vi "MonitoringOK7Param-moche.vi"() -> ()   [LabVIEW 2013]
panel:
  in  "Envoi":bool
  in  "data in":string
  out "?":bool
  in  "Afficher caractères reçus":bool
  in  "Log":bool
  out "error out":errorcluster
  out "Caractères reçus":string
  in  "Mode":T1(ring)=enum."CRLF"
  in  "?":bool
  in  "Tab Control":T2(tab)
  out "Par2":dbl
  out "Par1":dbl
  out "Signal Camera     ->    Fronts détectés":dbl[](graph)
  out "Signal Camera    ->  original":dbl[](graph)
  out "Par3":dbl
  out "Par 4":dbl
  out "Par 5":dbl
  out "Par 6":dbl
  out "Par 7":dbl
  in  "PID 3.3":dbl
  in  "PID 3.2":dbl
  in  "PID Direction":dbl
  in  "ABS":bool
  out "?":bool
  in  "PID vitesse":bool
  out "?":bool
  out "?":bool
  in  "PID 2.3":i8
  in  "PID 2.2":i8
  in  "PID Léger":i8
  in  "PID 1.3":i8
  in  "PID 1.2":i8
  in  "PID Fort":i8
  # "Fort"
  # "Léger"
  # "Droite"
  # "Gauche"
  # "Fin"
  # "Perte Ligne"
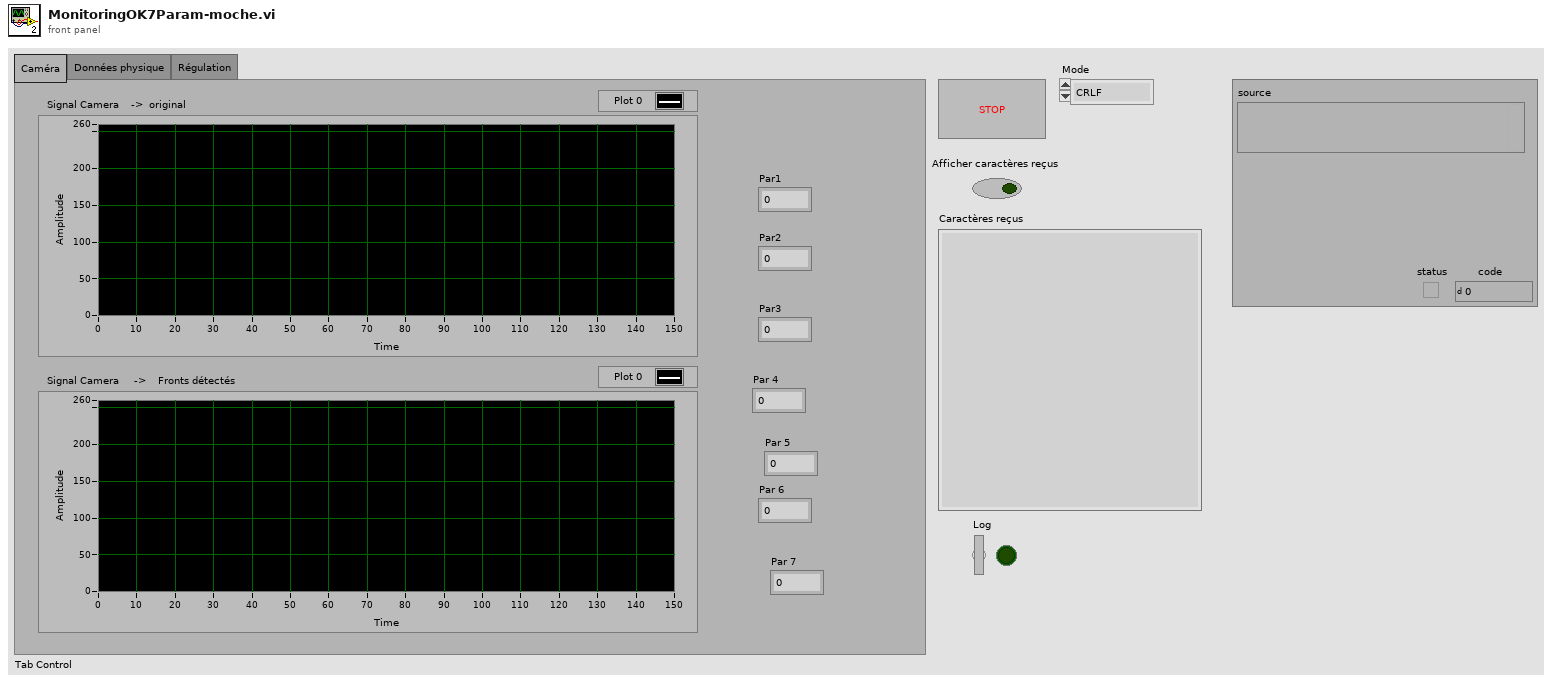
[diagram p1: front panel]
types:
  T1 = enum16{"Standard", "Buffered", "CRLF", "Immediate"}
  T2 = enum32{"Caméra", "Données physique", "Régulation"}
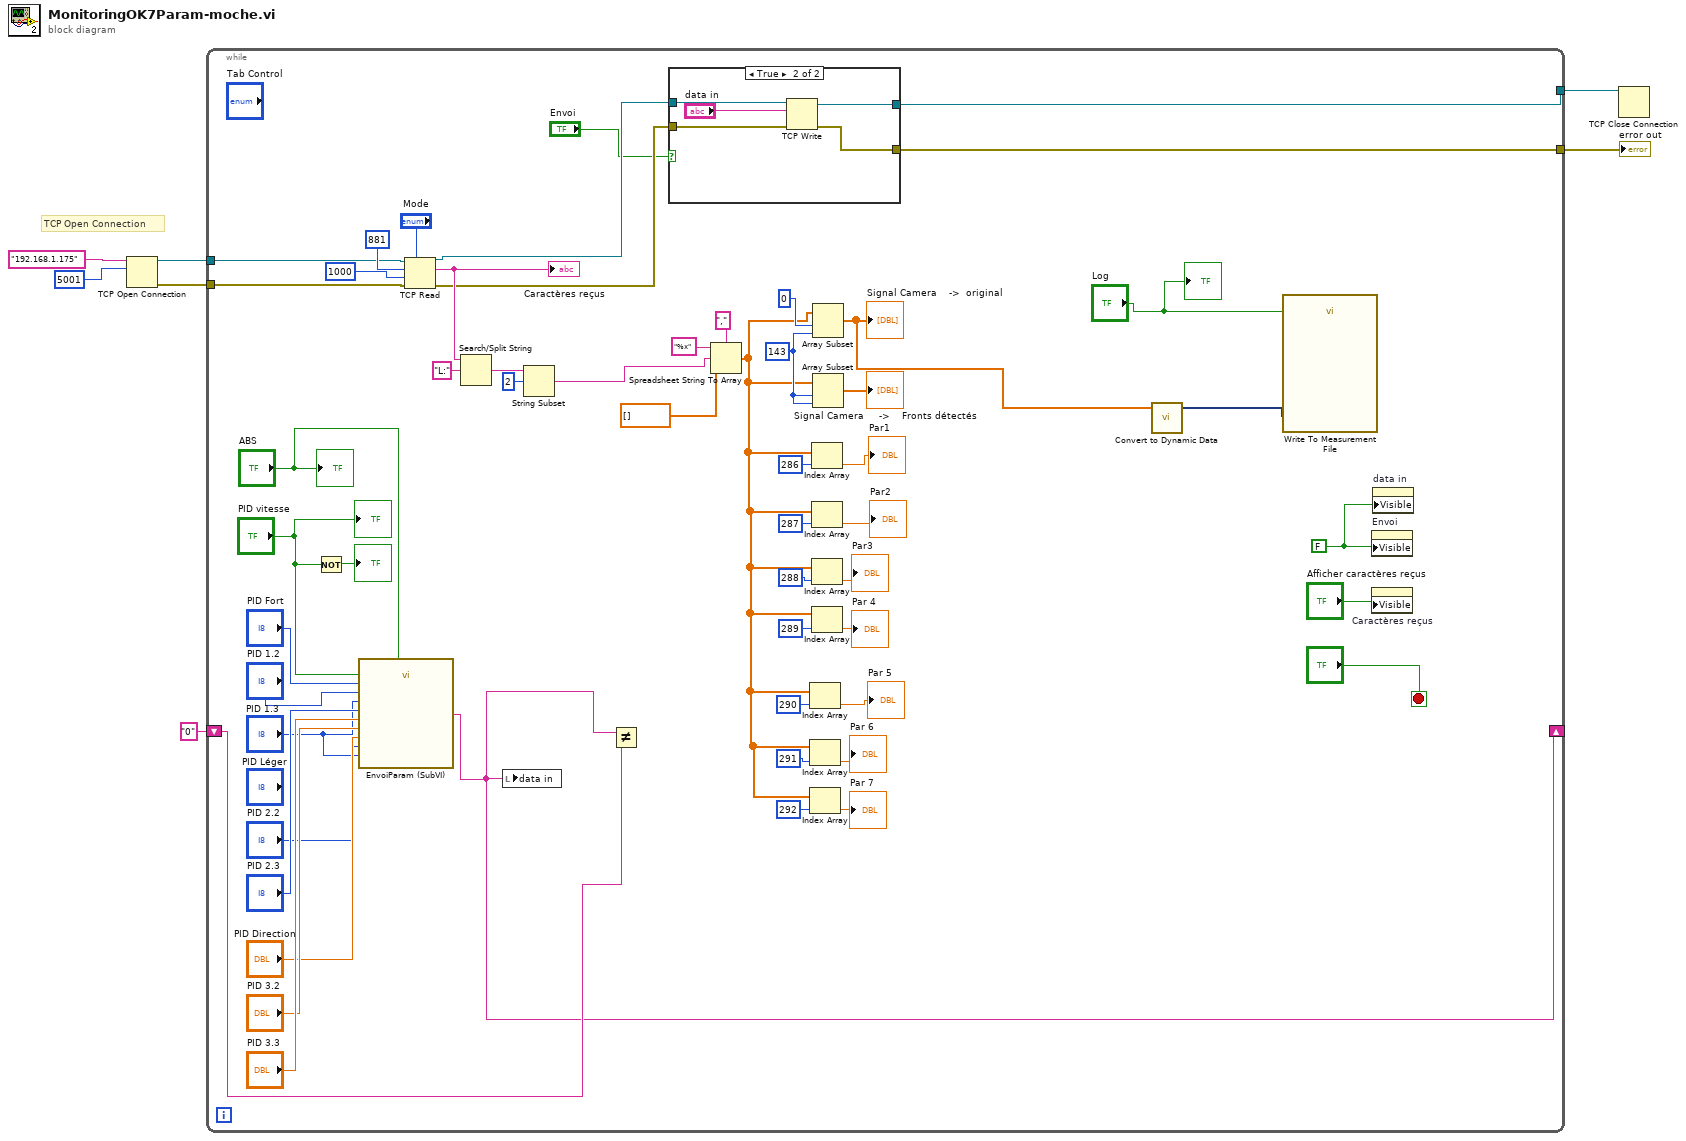
[diagram p0: block diagram]
diagram:
  # "TCP Open Connection"
  n1 = TCP Open Connection(address="192.168.1.175", remote port or service name=u16 5001) -> (connection ID=w5:refnum<k5>, error out=w4:errorcluster)  [unwired: 3 in]
  n2 = while {
    tunnel: w5 -> [w42]
    tunnel: w4 -> [w49]
    tunnel: [w40] -> w3
    tunnel: [w38] -> w2
    shift-right: [w25] -> _
    shift-left: "0" -> [w35]
    stop <- "?" stop-if-true
    w36 = FALSE
    w48 = 143 ("length")
    n3 = Not(x="PID vitesse") -> (.not. x?=→"?":bool)
    n4 = call "EnvoiParam (SubVI).vi"("PID 3.3"="PID 3.3", "PID 3.2"="PID 3.2", "PID Direction"="PID Direction", "PID 2.3"="PID 2.3", "PID 2.2"="PID 2.2", "PID Léger"="PID 1.3", "PID 1.3"="PID 1.3", "PID 1.2"="PID 1.2", "PID Fort"="PID Fort", "PID vitesse"="PID vitesse", "ABS"="ABS") -> ("String"=w25:string)
    n5 = TCP Read(connection ID=w42, bytes to read=881, error in (no error)=w49, 7:"Mode", 9:1000 ("timeout ms (25000)")) -> (connection ID out=w41:refnum<k5>, data out=w57:string, error out=w39:errorcluster)
    "Caractères reçus" <- w57
    n6 = Search/Split String(string=w57, search string/char (-)="L:") -> (match + rest of string=w55:string)  [unwired: 1 in, 2 out]
    n7 = local write "data in"(w25) -> ()
    n8 = String Subset(string=w55, offset (0)=2) -> (substring=w56:string)  [unwired: 1 in]
    n9 = Not Equal?(x=w25, y=w35) -> ()  [unwired: 1 out]
    n10 = case shown="True" "Envoi" {
      tunnel: w41 -> [w64 w69]
      tunnel: [w64 w68] -> w40
      tunnel: w39 -> [w63 w67]
      tunnel: [w63 w66] -> w38
      frame False {
      }
      frame True {
        n11 = TCP Write(connection ID=w69, data in="data in", error in (no error)=w67) -> (connection ID out=w68:refnum<k5>, error out=w66:errorcluster)  [unwired: 1 in, 1 out]
      }
    }
    n12 = Spreadsheet String To Array(delimiter (Tab)=",", format string="%x", spreadsheet string=w56, array type (2D Dbl)=dbl[] []) -> (array=w11:dbl[])
    n13 = Index Array(array=w11, index=290) -> (element=→"Par 5":dbl)
    n14 = Index Array(array=w11, index=291) -> (element=→"Par 6":dbl)
    n15 = Index Array(array=w11, index=292) -> (element=→"Par 7":dbl)
    n16 = Index Array(array=w11, index=286) -> (element=→"Par1":dbl)
    n17 = Index Array(array=w11, index=287) -> (element=→"Par2":dbl)
    n18 = Index Array(array=w11, index=288) -> (element=→"Par3":dbl)
    n19 = Index Array(array=w11, index=289) -> (element=→"Par 4":dbl)
    n20 = Array Subset(array=w11, index=0, length=w48) -> (w47:dbl[])
    "Signal Camera    ->  original" <- w47
    n21 = Array Subset(array=w11, index=w48, length=w48) -> (→"Signal Camera     ->    Fronts détectés":dbl[])
    n22 = call "Convert to Dynamic Data"("Array"=w47) -> ("Dynamic Data Type"=w45:dynamicdata)  [unwired: 3 in]
    n23 = call "Write To Measurement File"("Signals"=w45, "Enable"="Log") -> ()  [unwired: 15 in, 3 out]
    n24 = property on="Envoi" class="Bool (strict)"("Visible"=w36) -> ()  [unwired: 2 in, 2 out]
    n25 = property on="Caractères reçus" class="Str"("Visible"="Afficher caractères reçus") -> ()  [unwired: 2 in, 2 out]
    n26 = property on="data in" class="Str"("Visible"=w36) -> ()  [unwired: 2 in, 2 out]
    "?" <- "ABS"
    "?" <- "PID vitesse"
    "?" <- "Log"
  }
  "error out" <- w2
  n27 = TCP Close Connection(connection ID=w3) -> ()  [unwired: 2 in, 2 out]
